vi "UpdateNumberOfErrors.vi"(8 "error in (no error)":errorcluster, 10 "NumberOfErrord":u32, 11 "TCP_serverGUI in":refnum<class "TCP_serverGUI.lvclass">) -> (0 "error out":errorcluster, 3 "TCP_serverGUI out":refnum<class "TCP_serverGUI.lvclass">)   [LabVIEW 2023, in "TCP_serverGUI.lvlib" / "TCP_serverGUI.lvclass"]
uses:
  TCP_serverGUI.lvclass
  TCP_serverGUI.lvclass/TCP_serverGUI.ctl
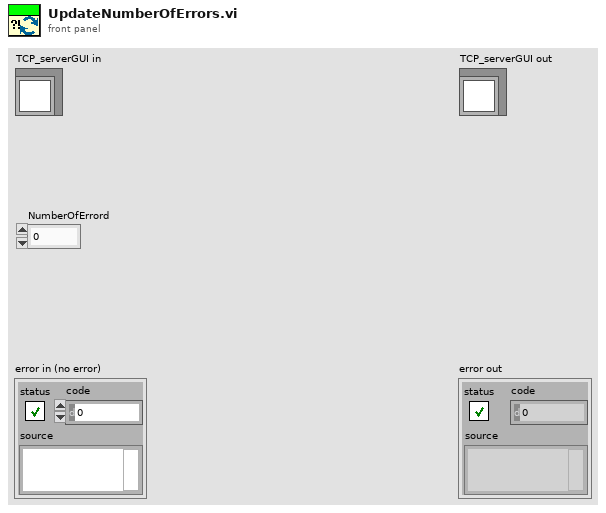
[diagram p1: front panel]
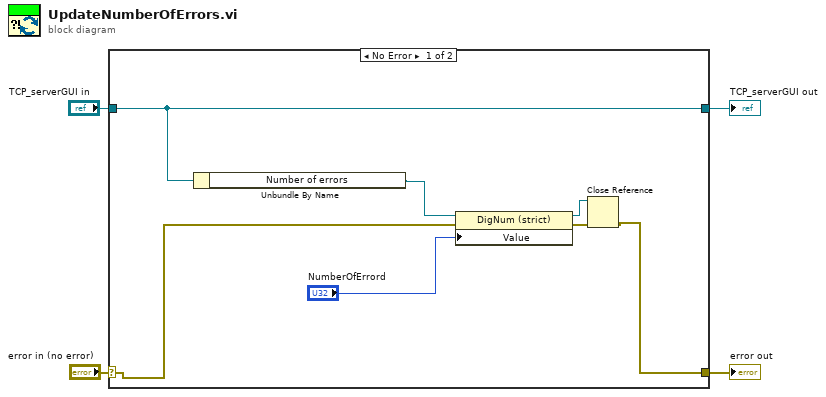
[diagram p0: block diagram]
diagram:
  n1 = case shown="No Error" "error in (no error)" {
    selector: "error in (no error)" -> [w6 w13]
    tunnel: [w5 w13] -> w3
    tunnel: [w11 w12] -> w1
    tunnel: "TCP_serverGUI in" -> [w11 w12]
    frame No Error {
      n2 = Unbundle By Name(w11) -> ("Number of errors"=w10:refnum<vi>)
      n3 = property class="DigNum (strict)"(reference=w10, error in=w6, "Value"="NumberOfErrord") -> (reference out=w8:refnum<vi>, error out=w9:errorcluster)
      n4 = Close Reference(reference=w8, error in (no error)=w9) -> (error out=w5:errorcluster)
    }
    frame Error {
    }
  }
  "error out" <- w3
  "TCP_serverGUI out" <- w1
